vi "Intake Controller.vi"(8 "error in":errorcluster) -> ()   [LabVIEW 2025]
doc: "This VI executes continuously carrying out the current operation and responding to updates or new operations. It will often contain the timing or control code that is difficult to place directly in TeleOp. This VI generally opens all sensors and motors and isolates the rest of the robot code from knowing how the operations are carried out."
uses:
  <vilib>/Rock Robotics/WPI/Framework/Completion Status.ctl
  Intake Setpoints.ctl
  Intake Operations.ctl
  <vilib>/Rock Robotics/WPI/ThirdParty/REV Robotics/REVLib/Typedef/SPARK Feed Forward Gains.ctl
  <vilib>/Rock Robotics/WPI/ThirdParty/REV Robotics/REVLib/Typedef/Spark MAX Idle Mode.ctl
  <vilib>/Rock Robotics/WPI/ThirdParty/REV Robotics/REVLib/Typedef/Spark MAX Control Type.ctl
  07c42978-d4ee-4343-8a12-b10232caffd9.vi
  <vilib>/Rock Robotics/WPI/ThirdParty/REV Robotics/REVLib/SubVI/Public/SPARK Open Brushless.vi
  <vilib>/Rock Robotics/WPI/ThirdParty/REV Robotics/REVLib/SubVI/Public/SPARK Configure Basic Idle Mode.vi
  <vilib>/Rock Robotics/WPI/ThirdParty/REV Robotics/REVLib/SubVI/Public/SPARK Configure Encoder Conversion Factors.vi
  <vilib>/Rock Robotics/WPI/ThirdParty/REV Robotics/REVLib/SubVI/Public/SPARK Configure Power Smart Current Limit.vi
  <vilib>/Rock Robotics/WPI/ThirdParty/REV Robotics/REVLib/SubVI/Public/SPARK Get Encoder Status Velocity.vi
  <vilib>/Rock Robotics/Network Tables/NT Write Boolean.vi
panel:
  out "Waveform Chart":T1(graph)
  in  "PID Gains":T3={{"P Gain"=3.0000000000000004e-05, "I Gain"=0.0, "D Gain"=0.0}, "Feed Forward Gains"={"kV"=0.00186, "kS"=0.0, "kA"=0.0, "kG"=0.0, "kCos"=0.0, "kCosRatio"=0.0}, "I Zone"=0.0, "Min Output"=-1.0, "Max Output"=1.0}
  in  "Cycle count":dbl=25.0
  in  "Interactive Values":T4
  out "Current\nCmd":string="Started at  00:20:52.642\nDefault: Reserve,  S 0.0, D 0.000000"
  in  "Buttons":cluster{"Execute Cmd":bool, "Abort Cmd":bool}
  out "Command Timing":cluster{"Start Time (ms)":u32, "Iterations":i32}={"Start Time (ms)"=900880, "Iterations"=0}
  out "Status":T6
  # "Interactive Command: You may fill in the settings for a command\nand schedule it with the Execute button. You can observe and abort\nany command while fine tuning the code for the controller."
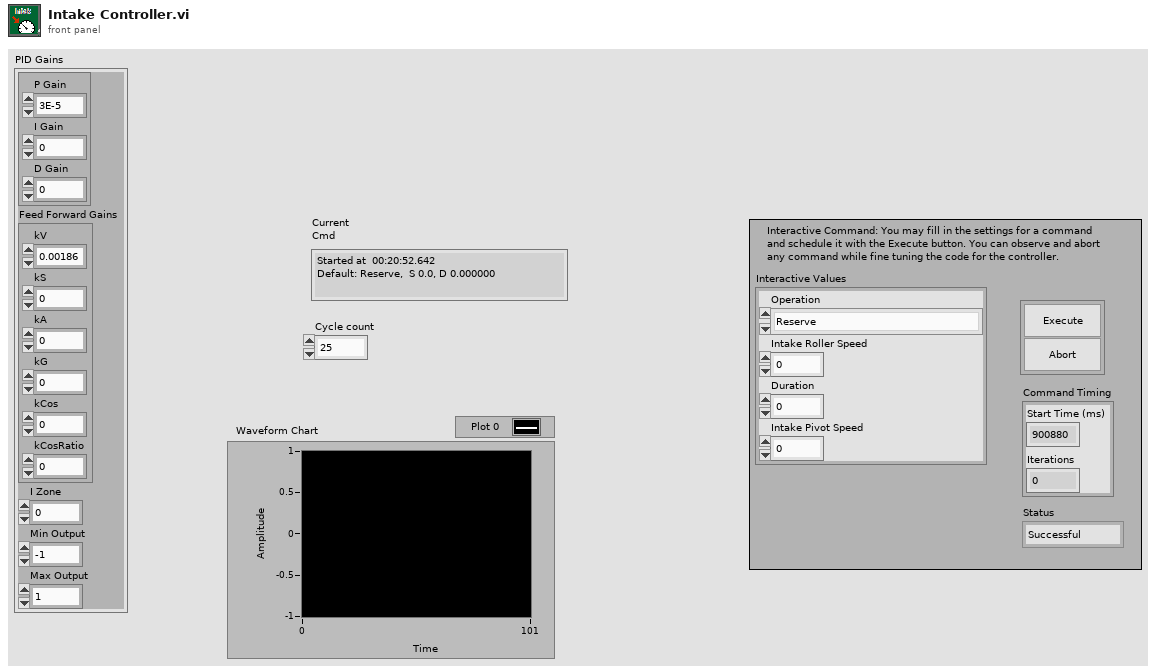
[diagram p1: front panel]
types:
  T1 = cluster{"Sensor Velocity":dbl, "Intake Roller Speed":dbl}
  T2 = typedef "SPARK Feed Forward Gains.ctl" = cluster{"kV":dbl, "kS":dbl, "kA":dbl, "kG":dbl, "kCos":dbl, "kCosRatio":dbl}
  T3 = cluster{cluster{"P Gain":dbl, "I Gain":dbl, "D Gain":dbl}, "Feed Forward Gains":T2, "I Zone":dbl, "Min Output":dbl, "Max Output":dbl}
  T4 = typedef "Intake Setpoints.ctl" = cluster{"Operation":T5, "Intake Roller Speed":dbl, "Duration":dbl, "Intake Pivot Speed":dbl}
  T5 = typedef "Intake Operations.ctl" = enum16{"Reserve", "Read Current", "Immediate", "Auto"}
  T6 = typedef "Completion Status.ctl" = enum16{"Successful", "Aborted", "Incomplete"}
  T7 = typedef "Spark MAX Idle Mode.ctl" = enum16{"Coast", "Brake"}
  T8 = typedef "WPI_MotorControlDeviceRef.ctl" = cluster{"DeviceStatus":errorcluster, "Type":T9, "PWM":cluster{"PWM Channel":T10, "DeadBand":T11}, "CAN":cluster{"Device Number":u8, "SetOutput VI Ref":variant, "GetOutput VI Ref":variant, "Enable VI Ref":variant, "Disable VI Ref":variant, "Data":variant}, "Invert":bool, "DIO PWM":cluster{"PWM \"Enable\" Channel":T10, "DIOChannel":T12, "PWM Rate":dbl}}
  T9 = typedef "WPI_MotorControlType.ctl" = enum16{"PWM", "CAN", "DIO PWM"}
  T10 = typedef "FPGA_DIOPWMChannel.ctl" = enum8{"PWM 0", "PWM 1", "PWM 2", "PWM 3", "PWM 4", "PWM 5", "PWM 6", "PWM 7", "PWM 8", "PWM 9", "PWM MXP 0", "PWM MXP 1", "PWM MXP 2", "PWM MXP 3", "PWM MXP 4", "PWM MXP 5", "PWM MXP 6", "PWM MXP 7", "PWM MXP 8", "PWM MXP 9", "Invalid"}
  T11 = typedef "WPI_PWMDeadband.ctl" = cluster{"Name":string, "maxPositivePwm":i32, "minPositivePwm":i32, "centerPwm":i32, "maxNegativePwm":i32, "minNegativePwm":i32, "angularRange":u16}
  T12 = typedef "FPGA_DIOChannel.ctl" = enum8{"DIO 0", "DIO 1", "DIO 2", "DIO 3", "DIO 4", "DIO 5", "DIO 6", "DIO 7", "DIO 8", "DIO 9", "DIO MXP 0", "DIO MXP 1", "DIO MXP 2", "DIO MXP 3", "DIO MXP 4", "DIO MXP 5", "DIO MXP 6", "DIO MXP 7", "DIO MXP 8", "DIO MXP 9", "DIO MXP 10", "DIO MXP 11", "DIO MXP 12", "DIO MXP 13", "DIO MXP 14", "DIO MXP 15", "SPI Port CS1", "SPI Port CS2", "SPI Port CS3", "SPI Port MISO", "SPI Port MOSI", "Invalid"}
  T13 = typedef "Command Status Info.ctl" = cluster{"Name":string, "Status":T6, "notifier out":T14}
  T14 = typedef "Completion Notifier.ctl" = refnum<notifier>
  T15 = cluster{"Current Command":T4, "Command Timing":cluster{"Start Time (ms)":u32, "Iterations":i32}, "Command Arguments":cluster{"Command Info":T13, "Description":string, "Default Command":T4, "queue out":refnum<queue>, "Subsystem Name":string}}
  T16 = typedef "Spark MAX Control Type.ctl" = enum16{"Percent VBus", "Voltage", "Velocity", "Position", "Smart Motion", "Current", "Smart Velocity", "MAXMotion Position", "MAXMotion Velocity"}
  T17 = typedef "WPI_DriverStationRobotMode2.ctl" = enum16{"Autonomous Disabled", "Autonomous Enabled", "Teleop Disabled", "Teleop Enabled", "Disconnected", "Finish", "Test Disabled", "Test Enabled", "Emergency Stopped"}
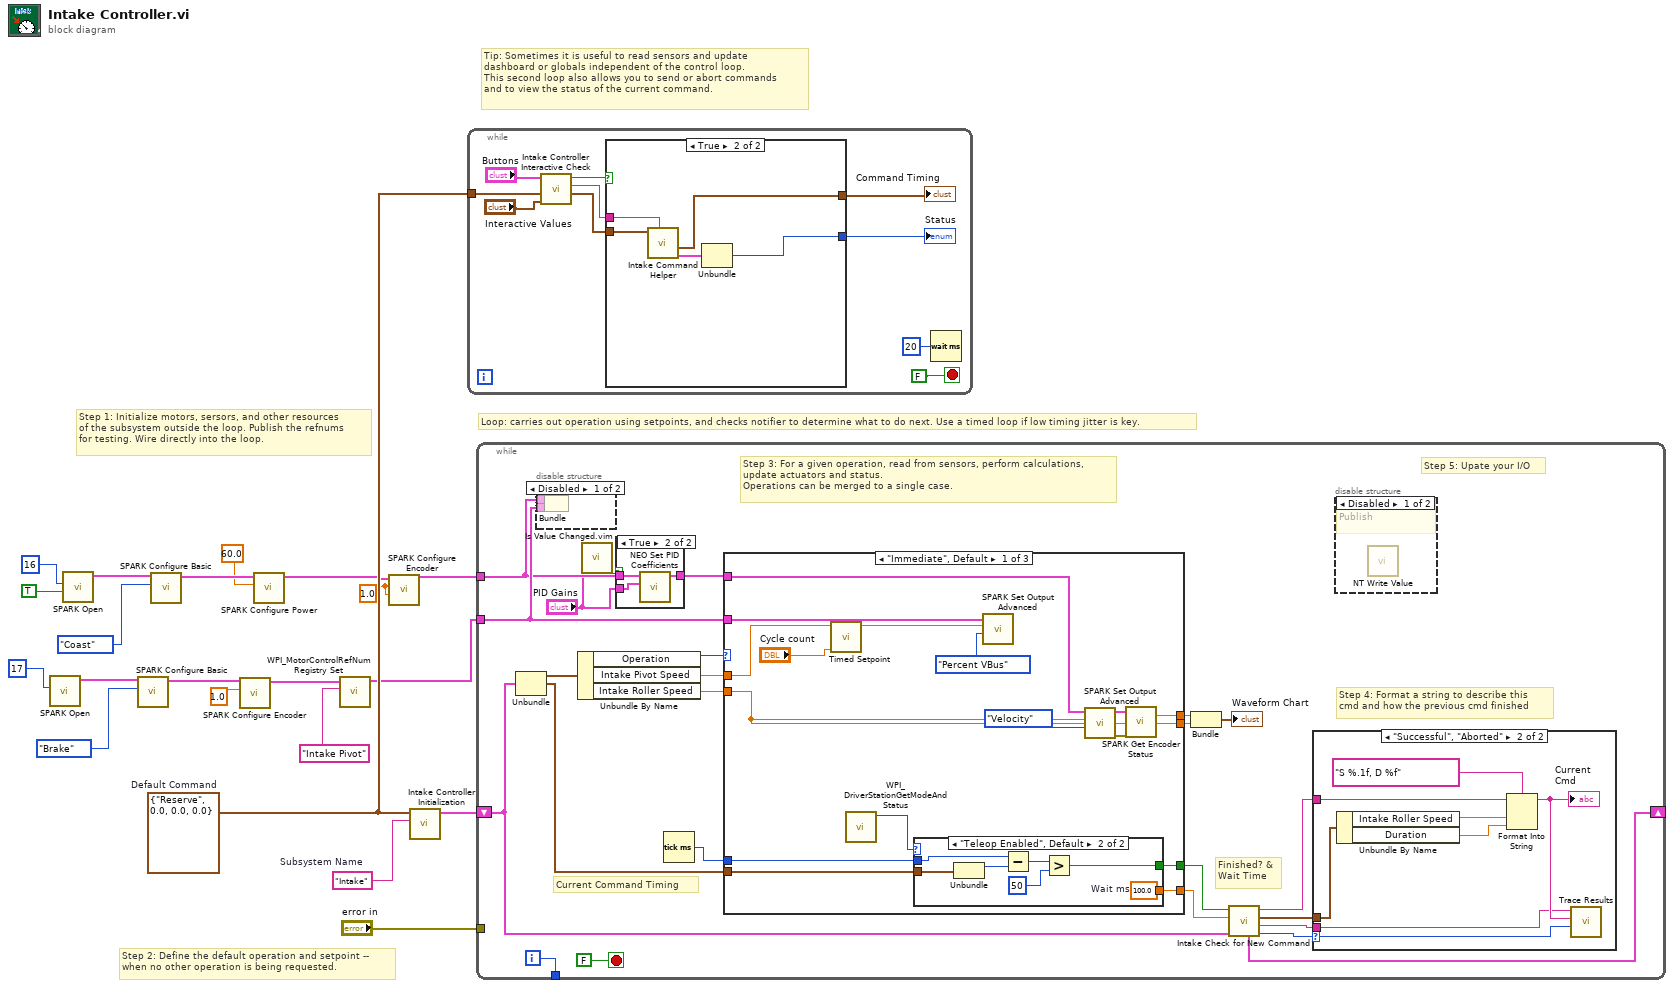
[diagram p0: block diagram]
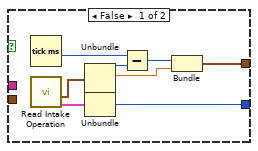
[diagram p2: hidden frame]
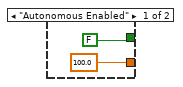
[diagram p7: hidden frame]
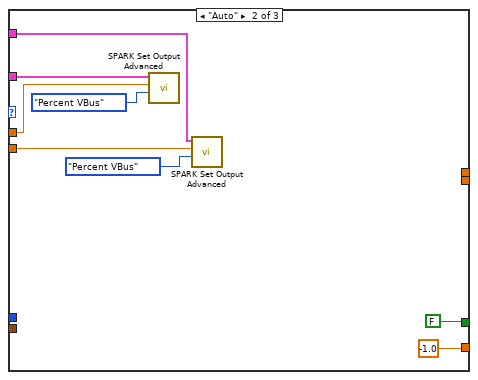
[diagram p8: hidden frame]
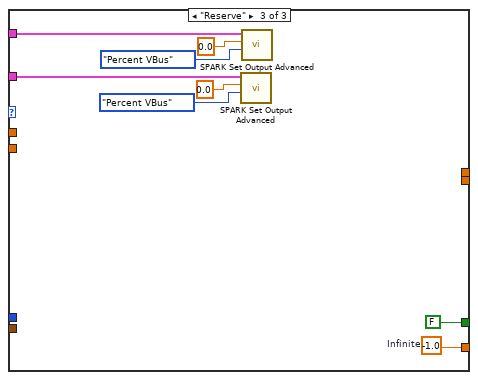
[diagram p9: hidden frame]
diagram:
  w1 = 1.0 ("Position Conversion Factor")
  w18 = T4 {"Operation"=enum."Reserve", "Intake Roller Speed"=0.0, "Duration"=0.0, "Intake Pivot Speed"=0.0}  # Default Command
  w19 = "Intake"  # Subsystem Name
  # "Tip: Sometimes it is useful to read sensors and update\ndashboard or globals independent of the control loop.\nThis second loop also allows you to send or abort commands\nand to view the status of the current command."
  # "Step 2: Define the default operation and setpoint --\nwhen no other operation is being requested."
  # "Step 1: Initialize motors, sersors, and other resources\nof the subsystem outside the loop. Publish the refnums\nfor testing. Wire directly into the loop."
  # "Loop: carries out operation using setpoints, and checks notifier to determine what to do next. Use a timed loop if low timing jitter is key."
  n1 = call-poly <vilib>:"SPARK Open.vi"("Device Number"=u8 17) -> ("MotorControlDeviceRef"=w12:T8)  [unwired: 9 in, 1 out]
  n2 = call-poly <vilib>:"SPARK Open.vi"("Invert"=TRUE, "Device Number"=u8 16) -> ("MotorControlDeviceRef"=w15:T8)  [unwired: 8 in, 1 out]
  n3 = call-poly <vilib>:"SPARK Configure Basic.vi"("Idle Mode"=Spark_MAX_Idle_Mode."Brake", "MotorControlDeviceRef in"=w12) -> ("MotorControlDeviceRef out"=w8:T8)  [unwired: 8 in, 1 out]
  n4 = call-poly <vilib>:"SPARK Configure Basic.vi"("Idle Mode"=Spark_MAX_Idle_Mode."Coast", "MotorControlDeviceRef in"=w15) -> ("MotorControlDeviceRef out"=w5:T8)  [unwired: 8 in, 1 out]
  n5 = call-poly <vilib>:"SPARK Configure Encoder.vi"("Position Conversion Factor"=1.0, "MotorControlDeviceRef in"=w8) -> ("MotorControlDeviceRef out"=w7:T8)  [unwired: 8 in, 1 out]
  n6 = call-poly <vilib>:"SPARK Configure Power.vi"("Primay Current Limit (80A)"=60.0, "MotorControlDeviceRef in"=w5) -> ("MotorControlDeviceRef out"=w3:T8)  [unwired: 8 in, 1 out]
  n7 = call <vilib>:"WPI_MotorControlRefNum Registry Set.vi"("refnum name"="Intake Pivot", "MotorControlDevRef"=w7) -> ("MotorControlDevRef"=w10:T8)  [unwired: 8 in, 1 out]
  n8 = call-poly <vilib>:"SPARK Configure Encoder.vi"("Velocity Conversion Factor"=w1, "Position Conversion Factor"=w1, "MotorControlDeviceRef in"=w3) -> ("MotorControlDeviceRef out"=w2:T8)  [unwired: 7 in, 1 out]
  n9 = call "Intake Controller Initialization.vi"("Subsystem Name"=w19, "Default Command"=w18) -> ("Current Command"=w20:T15)  [unwired: 9 in]
  n10 = while {
    tunnel: w18 -> [w28]
    stop <- FALSE stop-if-true
    n11 = call "Intake Controller Interactive Check.vi"("Interactive Command in"="Interactive Values", "Default Command"=w28, "Buttons"="Buttons") -> ("Interactive Command out"=w25:T4, "Trace String"=w26:string, "Schedule"=w27:bool)  [unwired: 6 in]
    n12 = case shown="True" w27 {
      tunnel: [w39 w44] -> w24
      tunnel: w25 -> [_ w42]
      tunnel: [w35 w40] -> w23
      tunnel: w26 -> [_ w43]
      frame False {
        n13 = Tick Count (ms)() -> (millisecond timer value=w34:u32)
        n14 = call "Read Intake Operation.vi"() -> ("Command Info"=w32:T13, "SubSystem Data"=w33:T4)  [unwired: 9 in, 1 out]
        n15 = Unbundle(w33) -> ("Operation"=w38:T5, "Intake Roller Speed"=w36:dbl)  [unwired: 2 out]
        n16 = Unbundle(w32) -> ("Status"=w39:T6)  [unwired: 2 out]
        n17 = Subtract(x=w34, y=w38) -> (x-y=w37:u32)
        n18 = Bundle(w37, "Intake Roller Speed"=w36) -> (w35:cluster{u32, "Intake Roller Speed":dbl})  [unwired: 1 in]
      }
      frame True {
        n19 = call "Intake Command Helper.vi"("Description"=w43, "SubSystem Data"=w42) -> ("Command Info Out"=w41:T13, "Command Timing"=w40:cluster{"Start Time (ms)":u32, "Iterations":i32})  [unwired: 7 in, 1 out]
        n20 = Unbundle(w41) -> ("Status"=w44:T6)  [unwired: 2 out]
      }
    }
    "Status" <- w24
    "Command Timing" <- w23
    n21 = Wait (ms)(milliseconds to wait=u32 20) -> ()  [unwired: 1 out]
  }
  n22 = while {
    shift-right: [w62] -> _
    shift-left: w20 -> [w55]
    tunnel: [w67] -> _
    tunnel: "error in" -> [_]
    tunnel: w2 -> [w51]
    tunnel: w10 -> [w52]
    i -> [w67]
    stop <- FALSE stop-if-true
    # "Step 5: Upate your I/O"
    # "Step 4: Format a string to describe this\ncmd and how the previous cmd finished"
    # "Current Command Timing"
    # "Finished? &\nWait Time"
    # "Step 3: For a given operation, read from sensors, perform calculations,\nupdate actuators and status.\nOperations can be merged to a single case."
    n23 = Unbundle(w55) -> ("Current Command"=w66:T4, "Command Timing"=w63:cluster{"Start Time (ms)":u32, "Iterations":i32})  [unwired: 1 out]
    n24 = disable-structure shown="Disabled" {
      disable-tunnel: w52 -> [w70 _]
      disable-tunnel: w51 -> [w69 _]
      frame Disabled {
        n25 = Bundle("MotorControlDeviceRef out"=w69, "MotorControlDevRef"=w70) -> ()  [unwired: 1 in, 1 out]
      }
      frame Enabled {
      }
    }
    n26 = Unbundle By Name(w66) -> ("Operation"=w65:T5, "Intake Pivot Speed"=w53:dbl, "Intake Roller Speed"=w54:dbl)
    n27 = call "Is Value Changed.vim"("value"="PID Gains") -> ("changed or first call?"=w49:bool)
    n28 = case shown="True" w49 {
      tunnel: w51 -> [w71 w74]
      tunnel: [w71 w73] -> w50
      tunnel: "PID Gains" -> [_ w72]
      frame False {
      }
      frame True {
        n29 = call "NEO Set PID Coefficients.vi"("PID Gains"=w72, "MotorControlDeviceRef in"=w74) -> ("MotorControlDeviceRef out"=w73:T8)  [unwired: 6 in, 1 out]
      }
    }
    n30 = Tick Count (ms)() -> (millisecond timer value=w64:u32)
    n31 = case shown="\"Immediate\", Default" w65 {
      tunnel: [w98 -1.0 ("Infinite") w123] -> w60
      tunnel: [w95 FALSE ("ignore previous (F)") FALSE ("ignore previous (F)")] -> w61
      tunnel: w63 -> [w97 _ _]
      tunnel: w64 -> [w96 _ _]
      tunnel: w50 -> [w93 w114 w120]
      tunnel: w52 -> [w91 w111 w116]
      tunnel: w54 -> [w84 w113 _]
      tunnel: w53 -> [w90 w110 _]
      tunnel: [w84 _ _] -> w47
      tunnel: [w83 _ _] -> w46
      frame "Immediate", Default {
        n32 = call "Timed Setpoint.vi"("Cycle count"="Cycle count", "Setpoint In"=w90) -> ("Setpoint Out"=w89:dbl)  [unwired: 9 in]
        n33 = call <vilib>:"WPI_DriverStationGetModeAndStatus.vi"() -> ("Robot Mode"=w87:T17)  [unwired: 10 in, 1 out]
        n34 = case shown="\"Teleop Enabled\", Default" w87 {
          tunnel: [100.0 ("Wait ms") w107] -> w98
          tunnel: w97 -> [_ w103]
          tunnel: w96 -> [_ w101]
          tunnel: [FALSE w102] -> w95
          frame "Autonomous Enabled" {
          }
          frame "Teleop Enabled", Default {
            w107 = 100.0  # Wait ms
            n35 = Unbundle(w103) -> ("Start Time (ms)"=w106:u32)  [unwired: 1 out]
            n36 = Subtract(x=w101, y=w106) -> (x-y=w105:u32)
            n37 = Greater?(x=w105, y=u8 50 ("Left Motor")) -> (0:w102:bool)
          }
        }
        n38 = call <vilib>:"SPARK Set Output Advanced.vi"("Control Mode"=Spark_MAX_Control_Type."Percent VBus", "Setpoint"=w89, "MotorControlDevRef"=w91) -> ()  [unwired: 7 in, 2 out]
        n39 = call <vilib>:"SPARK Set Output Advanced.vi"("Control Mode"=Spark_MAX_Control_Type."Velocity", "Setpoint"=w84, "MotorControlDevRef"=w93) -> ("error out"=w86:errorcluster, "MotorControlDevRef"=w85:T8)  [unwired: 7 in]
        n40 = call-poly <vilib>:"SPARK Get Encoder Status.vi"("error in (no error)"=w86, "MotorControlDevRef in"=w85) -> ("Sensor Velocity"=w83:dbl)  [unwired: 6 in, 3 out]
      }
      frame "Auto" {
        n41 = call <vilib>:"SPARK Set Output Advanced.vi"("Control Mode"=Spark_MAX_Control_Type."Percent VBus", "Setpoint"=w110, "MotorControlDevRef"=w111) -> ()  [unwired: 7 in, 2 out]
        n42 = call <vilib>:"SPARK Set Output Advanced.vi"("Control Mode"=Spark_MAX_Control_Type."Percent VBus", "Setpoint"=w113, "MotorControlDevRef"=w114) -> ()  [unwired: 7 in, 2 out]
      }
      frame "Reserve" {
        w123 = -1.0  # Infinite
        n43 = call <vilib>:"SPARK Set Output Advanced.vi"("Control Mode"=Spark_MAX_Control_Type."Percent VBus", "Setpoint"=0.0, "MotorControlDevRef"=w116) -> ()  [unwired: 7 in, 2 out]
        n44 = call <vilib>:"SPARK Set Output Advanced.vi"("Control Mode"=Spark_MAX_Control_Type."Percent VBus", "Setpoint"=0.0, "MotorControlDevRef"=w120) -> ()  [unwired: 7 in, 2 out]
      }
    }
    n45 = Bundle("Sensor Velocity"=w46, "Intake Roller Speed"=w47) -> (→"Waveform Chart":T1)  [unwired: 1 in]
    n46 = call "Intake Check for New Command.vi"("Current Command"=w55, "Wait time (ms)"=w60, "Finished?"=w61) -> ("Completion"=w56:T6, "Subsystem Name"=w57:string, "Current Command"=w58:T4, "Initial Trace String"=w59:string, "NextCommand"=w62:T15)  [unwired: 4 in]
    n47 = case shown="\"Successful\", \"Aborted\"" w56 {
      selector: w56 -> [_ w82]
      tunnel: w59 -> [_ w78]
      tunnel: w58 -> [_ w79]
      tunnel: w57 -> [_ w75]
      frame "Incomplete", Default {
        # "Continuing current command"
      }
      frame "Successful", "Aborted" {
        # "Report and setup for next command"
        n48 = Unbundle By Name(w79) -> ("Intake Roller Speed"=w81:dbl, "Duration"=w76:dbl)
        n49 = Format Into String(format string="S %.1f, D %f", initial string=w78, w81, w76) -> (resulting string=w77:string)  [unwired: 1 in, 1 out]
        "Current\nCmd" <- w77
        n50 = call <vilib>:"Trace Results.vi"("Status of previous command"=w82, "Description"=w77, "Subsystem"=w75) -> ()  [unwired: 9 in]
      }
    }
    n51 = disable-structure shown="Disabled" {
      frame Disabled {
        # "Publish"
        n52 = call-poly <vilib>:"NT Write Value.vi"() -> ()  [unwired: 11 in, 1 out]
      }
      frame Enabled {
      }
    }
  }
